vi "test.logToTDMS.vi"() -> ()   [LabVIEW 2017]
uses:
  File/_FileName Rule.ctl
panel:
  out "File":path
  out "DataCount":i32
  in  "stop":bool
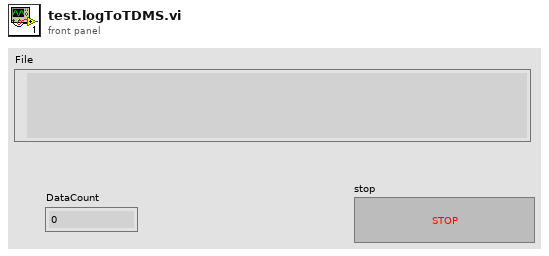
[diagram p1: front panel]
types:
  T1 = typedef "_FileName Rule.ctl" = cluster{"Rule":enum16{"Fixed File Name", "Indexed File Name", "TimeBased File Name"}, "Path":path, "filename":string}
  T2 = cluster{"FileNameRule":T1, "FileOperation":enum16{"open", "open or create", "create or replace", "create", "open (read-only)"}, "byte order (2:little-endian)":enum16{"big-endian, network order", "native, host order", "little-endian"}, "disable buffering? (T)":bool}
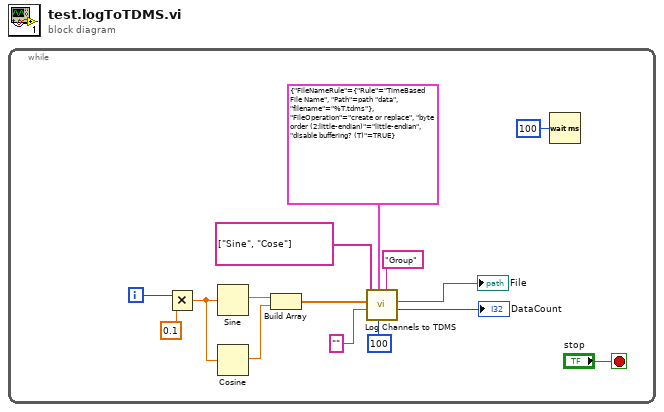
[diagram p0: block diagram]
diagram:
  n1 = while {
    i -> [w13]
    stop <- "stop" stop-if-true
    n2 = Multiply(x=w13, y=0.1) -> (x*y=w11:dbl)
    n3 = Sine(x=w11) -> (sin(x)=w9:dbl)
    n4 = Cosine(x=w11) -> (cos(x)=w8:dbl)
    n5 = Build Array(w9, w8) -> (w7:dbl[])
    n6 = call "Log Channels to TDMS.vi"("group name in (Group)"="Group", "Limit(-1)"=100, "NameRule"=T2 {"FileNameRule"={"Rule"=enum."TimeBased File Name", "Path"=path "data", "filename"="%T.tdms"}, "FileOperation"=enum."create or replace", "byte order (2:little-endian)"=enum."little-endian", "disable buffering? (T)"=TRUE}, "TimeChannel(\"\" Empty to Skip)"="" ("TimeChannel(\"\" Empty to Skip)"), "Array"=w7, "channel names"=string[] ["Sine", "Cose"]) -> ("DataCount"=→"DataCount":i32, "File"=→"File":path)  [unwired: 3 in, 1 out]
    n7 = Wait (ms)(milliseconds to wait=u32 100) -> ()  [unwired: 1 out]
  }
